vi "MQTT_ConnAck_Send.vi"(8 "error in (no error)":errorcluster, 10 "Conn Return Code":T1=enum."Connection refused: not authorized", 11 "connection ID":refnum<k5>) -> (0 "error out":errorcluster, 2 "ConnAck Message":u8[](array[numeric]) format="%x", 3 "connection ID out":refnum<k5>)   [LabVIEW 2020, in "MQTT_Functions.lvlib"]
uses:
  MQTT_Functions.lvlib
  Controls/MessageType.ctl
  Controls/Retain_Flag.ctl
  Controls/DUP_Flag.ctl
  Controls/QoS.ctl
  Controls/Connection_Return_Codes.ctl
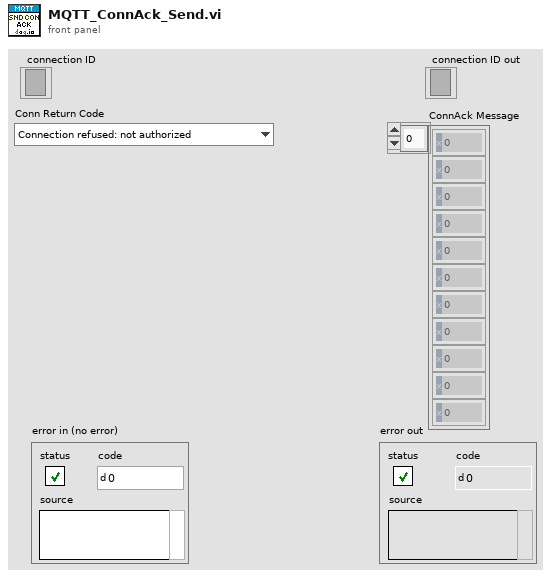
[diagram p1: front panel]
types:
  T1 = typedef "MQTT_Functions.lvlib/Connection_Return_Codes.ctl" = enum16{"Connection accepted", "Connection refused: unacceptable protocol version", "Connection refused: identifier rejected", "Connection refused: Server unavailable", "Connection refused: bad user name or password", "Connection refused: not authorized"}
  T2 = typedef "MQTT_Functions.lvlib/QoS.ctl" = enum8{"At most once", "At least once", "Exactly once", "Reserved"}
  T3 = typedef "MQTT_Functions.lvlib/DUP_Flag.ctl" = bool
  T4 = typedef "MQTT_Functions.lvlib/Retain_Flag.ctl" = bool
  T5 = typedef "MQTT_Functions.lvlib/MessageType.ctl" = enum32{"Reserved", "CONNECT", "CONNACK", "PUBLISH", "PUBACK", "PUBREC", "PUBREL", "PUBCOMP", "SUBSCRIBE", "SUBACK", "UNSUBSCRIBE", "UNSUBACK", "PINGREQ", "PINGRESP", "DISCONNECT", "Reserved2"}
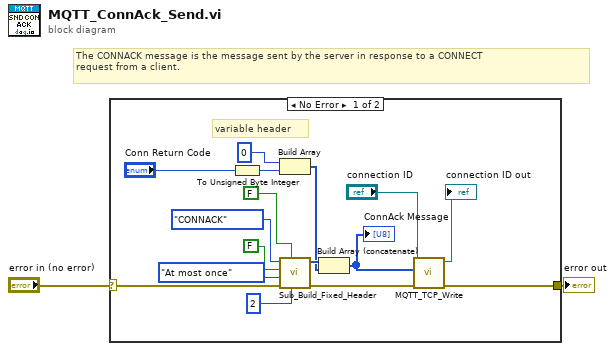
[diagram p0: block diagram]
diagram:
  # "The CONNACK message is the message sent by the server in response to a CONNECT\nrequest from a client."
  n1 = case shown="No Error" "error in (no error)" {
    selector: "error in (no error)" -> [w12 w19]
    tunnel: [w5 w19] -> w1
    frame No Error {
      # "variable header"
      n2 = To Unsigned Byte Integer(number="Conn Return Code") -> (unsigned 8bit integer=w9:u8)
      n3 = Build Array(u8 0 ("element"), w9) -> (w11:u8[])
      n4 = call "Sub_Build_Fixed_Header.vi"("Remaining Length"=u32 2, "Retain"=T4 FALSE, "error in (no error)"=w12, "QoS"=QoS."At most once", "DUP"=T3 FALSE, "MessageType"=MessageType."CONNACK") -> ("error out"=w6:errorcluster, "Fixed Header"=w17:u8[])  [unwired: 4 in]
      n5 = Build Array (concatenate)(w17, w11) -> (w7:u8[])
      "ConnAck Message" <- w7
      n6 = call "MQTT_TCP_Write.vi"("error in (no error)"=w6, "data in"=w7, "connection ID"="connection ID") -> ("error out"=w5:errorcluster, "connection ID out"=→"connection ID out":refnum<k5>)  [unwired: 6 in, 1 out]
    }
    frame Error {
    }
  }
  "error out" <- w1
